vi "main-top-level-example.vi"() -> ()   [LabVIEW 2024]
uses:
  controls/digital-output-cluster.ctl
  controls/thermocouple-input-cluster.ctl
  controls/analog-input-cluster.ctl
  controls/adam-5000-cmd-response.ctl
  controls/state-enum.ctl
  controls/adam-5000-all-chassis-data.ctl
  controls/adam-5000-all-module-datas.ctl
  controls/digitial-input-cluster.ctl
  controls/analog-output-cluster.ctl
  controls/adam-5000-chassis-cmd-ack.ctl
  controls/adam-5000-chassis-module-types.ctl
  controls/adam-5000-DO-user-input.ctl
  controls/adam-5000-status-indicator-references.ctl
  controls/adam-5000-serial-settings.ctl
panel:
  out "Program State":T1
  in  "Start ADAM":bool
  out "cmd-response":T3
  out "Status Indicators":T4
  in  "Debug Mode":bool
  out "1.Thermocouple Inputs (degC)":T5
  in  "5:Digital Outputs":T6
  in  "4:Digital Outputs":T6
  out "0:Analog Inputs":T7
  out "3:Thermocouple Inputs (degC)":T5
  in  "Chassis Settings":T8={"VISA resource name"="COM8", "baud rate (19200)"=19200, "Chassis ID"=1}
  out "Loop Time (mS)":u32
  out "Loop Counter":i32
  out "error IO":errorcluster
  out "error":errorcluster
  in  "exit":bool
  # "ADAM 5000 Controller"
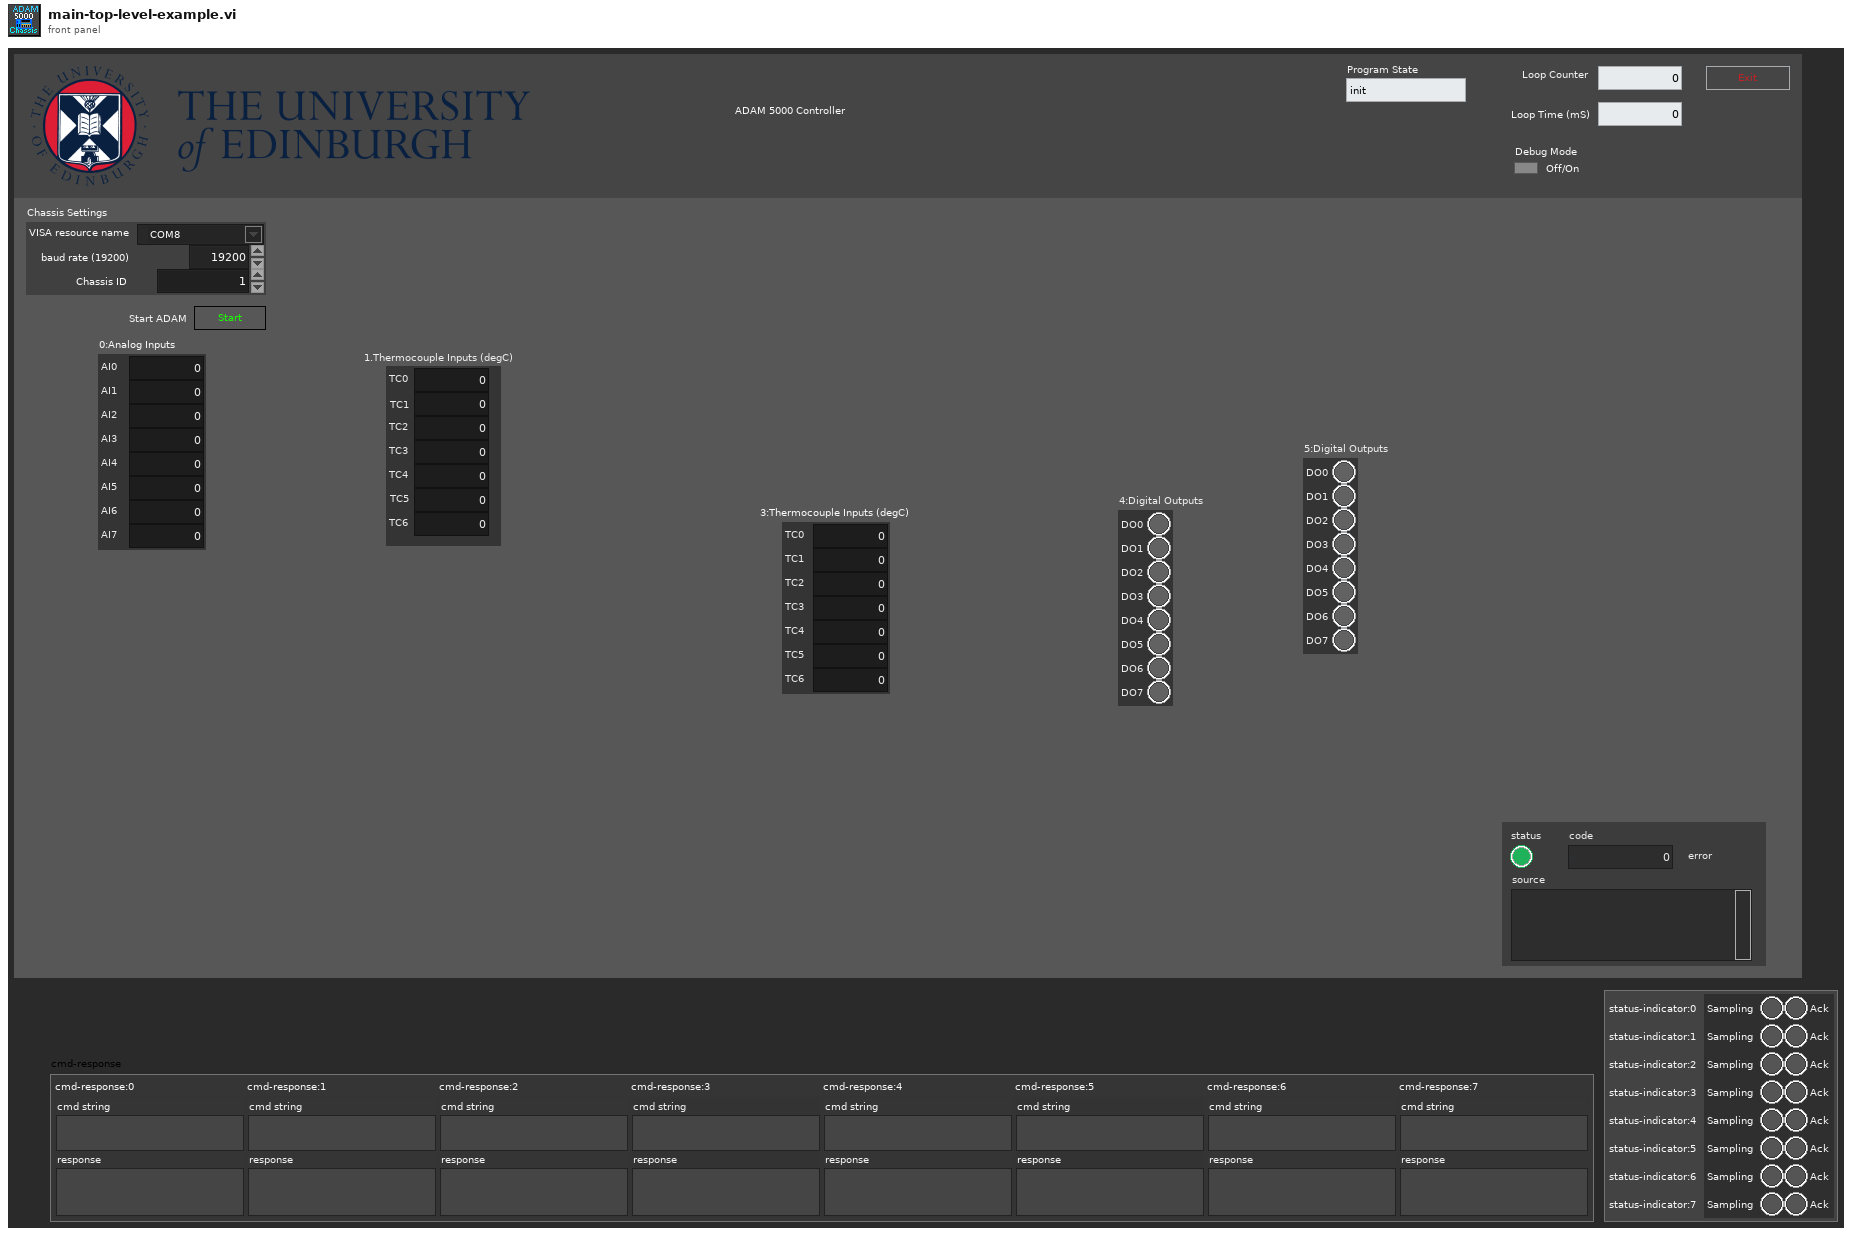
[diagram p1: front panel]
types:
  T1 = typedef "state-enum.ctl" = enum16{"init", "wait", "manual", "start", "run", "hold", "stop", "exit"}
  T2 = typedef "adam-5000-cmd-response.ctl" = cluster{"cmd string":string, "response":string}
  T3 = cluster{"cmd-response:0":T2, "cmd-response:1":T2, "cmd-response:2":T2, "cmd-response:3":T2, "cmd-response:4":T2, "cmd-response:5":T2, "cmd-response:6":T2, "cmd-response:7":T2}
  T4 = cluster{"status-indicator:0":cluster{"Sampling":bool, "Ack":bool}, "status-indicator:1":cluster{"Sampling":bool, "Ack":bool}, "status-indicator:2":cluster{"Sampling":bool, "Ack":bool}, "status-indicator:3":cluster{"Sampling":bool, "Ack":bool}, "status-indicator:4":cluster{"Sampling":bool, "Ack":bool}, "status-indicator:5":cluster{"Sampling":bool, "Ack":bool}, "status-indicator:6":cluster{"Sampling":bool, "Ack":bool}, "status-indicator:7":cluster{"Sampling":bool, "Ack":bool}}
  T5 = typedef "thermocouple-input-cluster.ctl" = cluster{"TC0":dbl, "TC1":dbl, "TC2":dbl, "TC3":dbl, "TC4":dbl, "TC5":dbl, "TC6":dbl}
  T6 = typedef "digital-output-cluster.ctl" = cluster{"DO0":bool, "DO1":bool, "DO2":bool, "DO3":bool, "DO4":bool, "DO5":bool, "DO6":bool, "DO7":bool}
  T7 = typedef "analog-input-cluster.ctl" = cluster{"AI0":dbl, "AI1":dbl, "AI2":dbl, "AI3":dbl, "AI4":dbl, "AI5":dbl, "AI6":dbl, "AI7":dbl}
  T8 = typedef "adam-5000-serial-settings.ctl" = cluster{"VISA resource name":refnum<visa-resource-name>, "baud rate (19200)":u32, "Chassis ID":u8}
  T9 = typedef "adam-5000-chassis-cmd-ack.ctl" = cluster{"cmd-response:0":T2, "cmd-response:1":T2, "cmd-response:2":T2, "cmd-response:3":T2, "cmd-response:4":T2, "cmd-response:5":T2, "cmd-response:6":T2, "cmd-response:7":T2}
  T10 = typedef "adam-5000-all-chassis-data.ctl" = cluster{"slot:0":T11, "slot:1":T11, "slot:2":T11, "slot:3":T11, "slot:4":T11, "slot:5":T11, "slot:6":T11, "slot:7":T11}
  T11 = typedef "adam-5000-all-module-datas.ctl" = cluster{"Digital Outputs":T6, "Digital Inputs":T12, "Analog Outputs":T13, "Analog Inputs":T7, "Thermocouple Inputs (degC)":T5}
  T12 = typedef "digitial-input-cluster.ctl" = cluster{"DI0":bool, "DI1":bool, "DI2":bool, "DI3":bool, "DI4":bool, "DI5":bool, "DI6":bool, "DI7":bool}
  T13 = typedef "analog-output-cluster.ctl" = cluster{"AO0":dbl, "AO1":dbl, "AO2":dbl, "AO3":dbl}
  T14 = enum16{"Digital Output", "Digital Input", "Analog Output", "Analog Input", "Thermocouple", "Power Relay", "empty"}
  T15 = enum8{"Enabled", "Disabled", "Disabled and Grayed Out"}
  T16 = typedef "adam-5000-status-indicator-references.ctl" = cluster{"status-indicator:0":refnum<vi>, "status-indicator:1":refnum<vi>, "status-indicator:2":refnum<vi>, "status-indicator:3":refnum<vi>, "status-indicator:4":refnum<vi>, "status-indicator:5":refnum<vi>, "status-indicator:6":refnum<vi>, "status-indicator:7":refnum<vi>}
  T17 = typedef "adam-5000-DO-user-input.ctl" = cluster{"0:Digital Outputs":T6, "1:Digital Outputs":T6, "2:Digital Outputs":T6, "3:Digital Outputs":T6, "4:Digital Outputs":T6, "5:Digital Outputs":T6, "6:Digital Outputs":T6, "7:Digital Outputs":T6}
  T18 = typedef "adam-5000-chassis-module-types.ctl" = cluster{"Slot 0: Module Type":enum16{"Digital Output", "Digital Input", "Analog Output", "Analog Input", "Thermocouple", "Power Relay", "empty"}, "Slot 1: Module Type":enum16{"Digital Output", "Digital Input", "Analog Output", "Analog Input", "Thermocouple", "Power Relay", "empty"}, "Slot 2: Module Type":enum16{"Digital Output", "Digital Input", "Analog Output", "Analog Input", "Thermocouple", "Power Relay", "empty"}, "Slot 3: Module Type":enum16{"Digital Output", "Digital Input", "Analog Output", "Analog Input", "Thermocouple", "Power Relay", "empty"}, "Slot 4: Module Type":enum16{"Digital Output", "Digital Input", "Analog Output", "Analog Input", "Thermocouple", "Power Relay", "empty"}, "Slot 5: Module Type":enum16{"Digital Output", "Digital Input", "Analog Output", "Analog Input", "Thermocouple", "Power Relay", "empty"}, "Slot 6: Module Type":enum16{"Digital Output", "Digital Input", "Analog Output", "Analog Input", "Thermocouple", "Power Relay", "empty"}, "Slot 7: Module Type":enum16{"Digital Output", "Digital Input", "Analog Output", "Analog Input", "Thermocouple", "Power Relay", "empty"}}
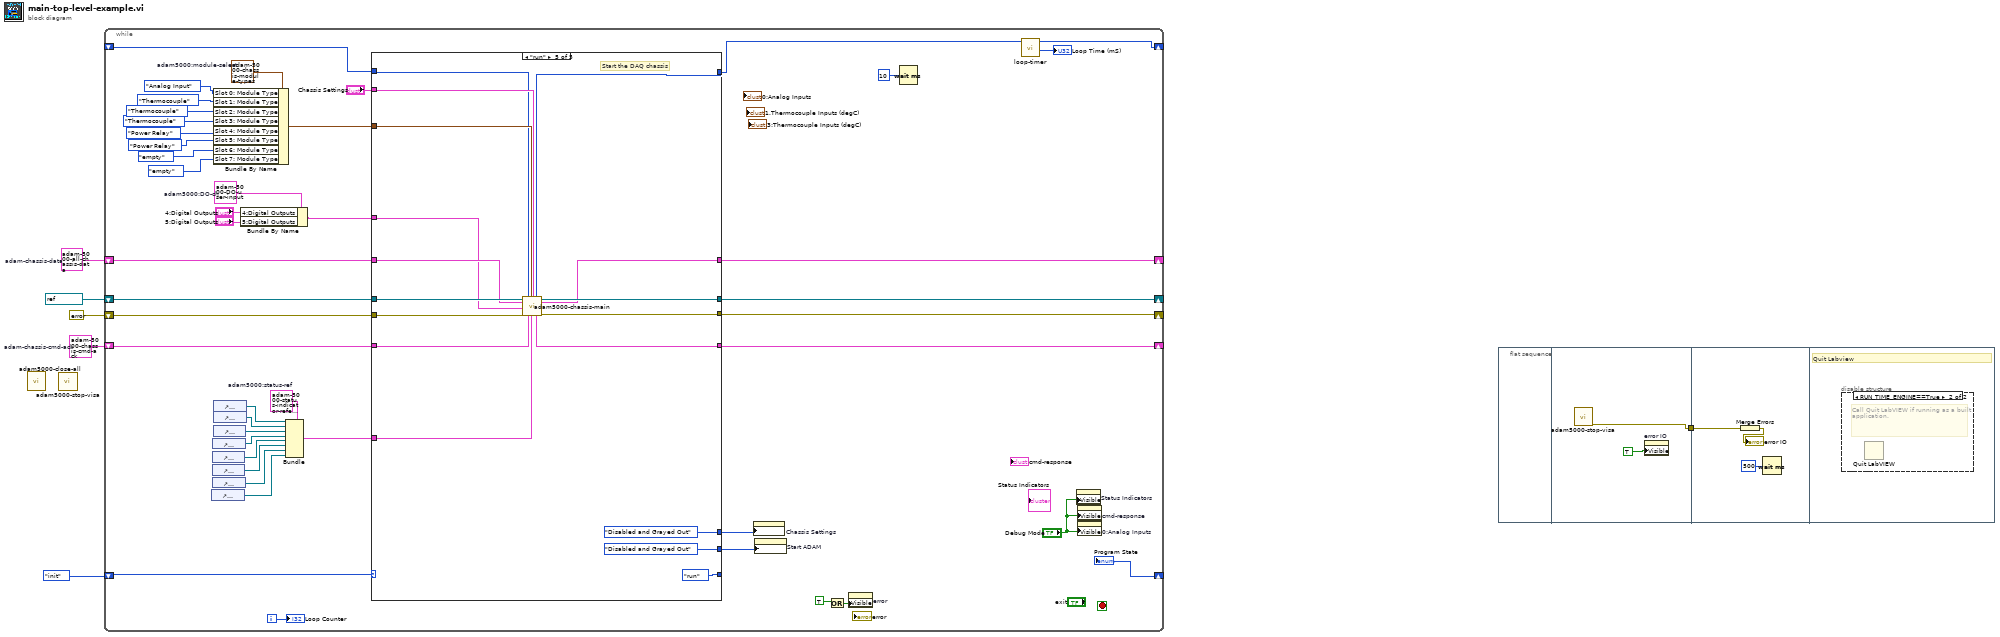
[diagram p0: block diagram]
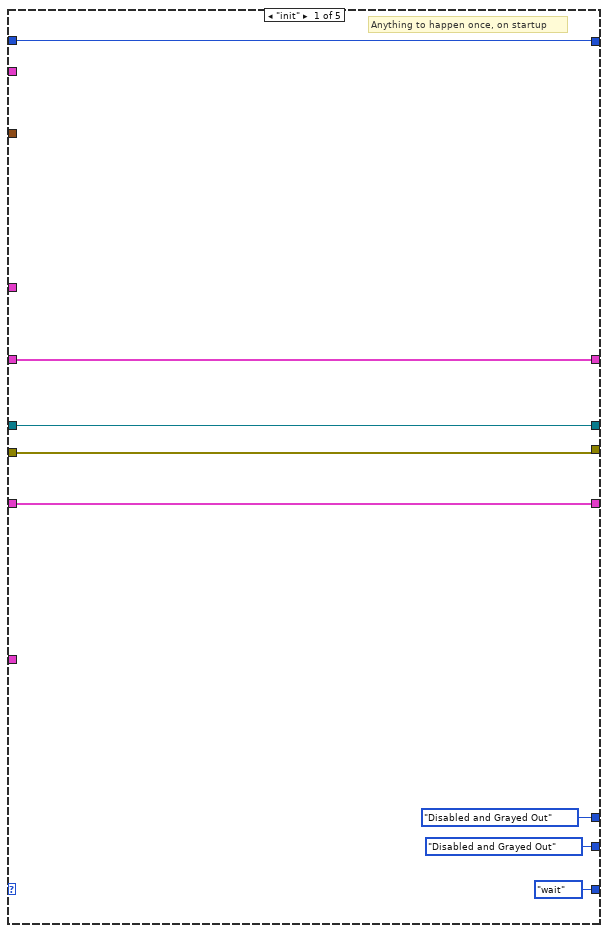
[diagram p3: hidden frame]
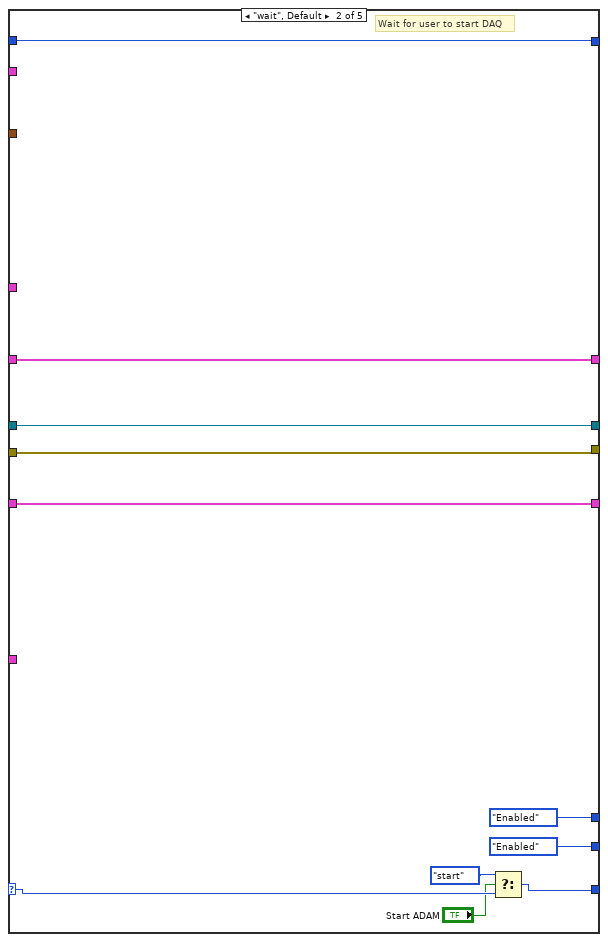
[diagram p4: hidden frame]
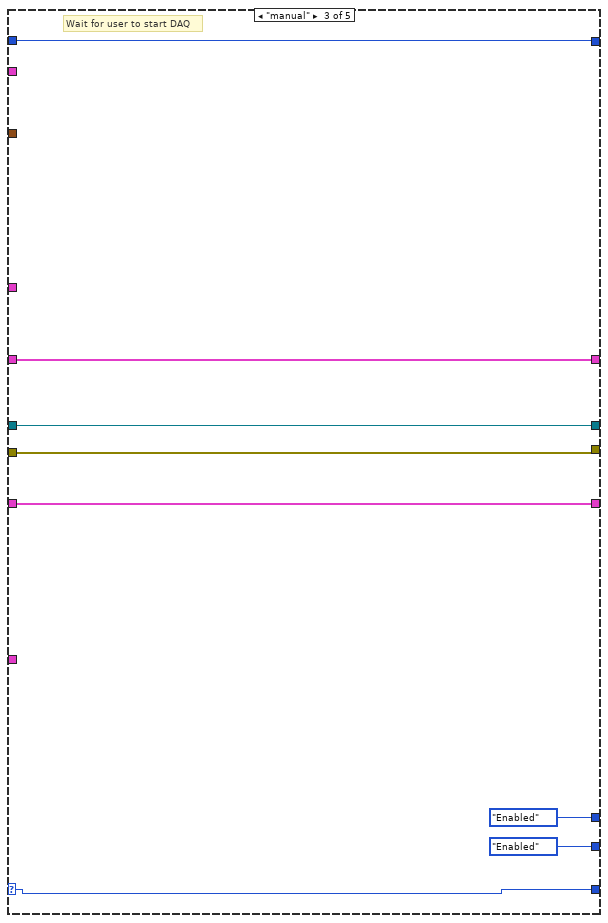
[diagram p5: hidden frame]
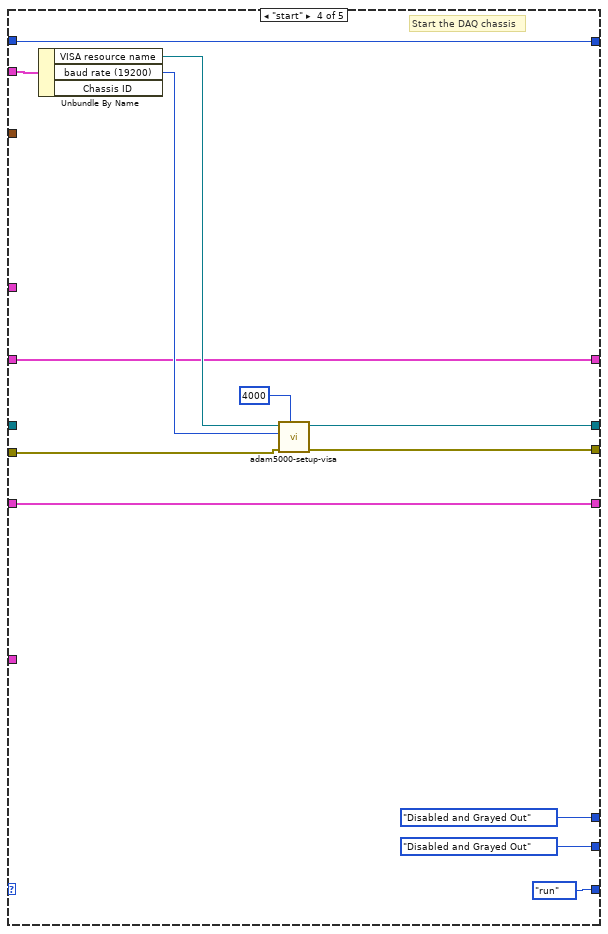
[diagram p6: hidden frame]
diagram:
  w1 = T9 {"cmd-response:0"={"cmd string"="", "response"=""}, "cmd-response:1"={"cmd string"="", "response"=""}, "cmd-response:2"={"cmd string"="", "response"=""}, "cmd-response:3"={"cmd string"="", "response"=""}, "cmd-response:4"={"cmd string"="", "response"=""}, "cmd-response:5"={"cmd string"="", "response"=""}, "cmd-response:6"={"cmd string"="", "response"=""}, "cmd-response:7"={"cmd string"="", "response"=""}}  # adam-chassis-cmd-ack
  w2 = T10 {"slot:0"={"Digital Outputs"={"DO0"=FALSE, "DO1"=FALSE, "DO2"=FALSE, "DO3"=FALSE, "DO4"=FALSE, "DO5"=FALSE, "DO6"=FALSE, "DO7"=FALSE}, "Digital Inputs"={"DI0"=FALSE, "DI1"=FALSE, "DI2"=FALSE, "DI3"=FALSE, "DI4"=FALSE, "DI5"=FALSE, "DI6"=FALSE, "DI7"=FALSE}, "Analog Outputs"={"AO0"=0.0, "AO1"=0.0, "AO2"=0.0, "AO3"=0.0}, "Analog Inputs"={"AI0"=0.0, "AI1"=0.0, "AI2"=0.0, "AI3"=0.0, "AI4"=0.0, "AI5"=0.0, "AI6"=0.0, "AI7"=0.0}, "Thermocouple Inputs (degC)"={"TC0"=0.0, "TC1"=0.0, "TC2"=0.0, "TC3"=0.0, "TC4"=0.0, "TC5"=0.0, "TC6"=0.0}}, "slot:1"={"Digital Outputs"={"DO0"=FALSE, "DO1"=FALSE, "DO2"=FALSE, "DO3"=FALSE, "DO4"=FALSE, "DO5"=FALSE, "DO6"=FALSE, "DO7"=FALSE}, "Digital Inputs"={"DI0"=FALSE, "DI1"=FALSE, "DI2"=FALSE, "DI3"=FALSE, "DI4"=FALSE, "DI5"=FALSE, "DI6"=FALSE, "DI7"=FALSE}, "Analog Outputs"={"AO0"=0.0, "AO1"=0.0, "AO2"=0.0, "AO3"=0.0}, "Analog Inputs"={"AI0"=0.0, "AI1"=0.0, "AI2"=0.0, "AI3"=0.0, "AI4"=0.0, "AI5"=0.0, "AI6"=0.0, "AI7"=0.0}, "Thermocouple Inputs (degC)"={"TC0"=0.0, "TC1"=0.0, "TC2"=0.0, "TC3"=0.0, "TC4"=0.0, "TC5"=0.0, "TC6"=0.0}}, "slot:2"={"Digital Outputs"={"DO0"=FALSE, "DO1"=FALSE, "DO2"=FALSE, "DO3"=FALSE, "DO4"=FALSE, "DO5"=FALSE, "DO6"=FALSE, "DO7"=FALSE}, "Digital Inputs"={"DI0"=FALSE, "DI1"=FALSE, "DI2"=FALSE, "DI3"=FALSE, "DI4"=FALSE, "DI5"=FALSE, "DI6"=FALSE, "DI7"=FALSE}, "Analog Outputs"={"AO0"=0.0, "AO1"=0.0, "AO2"=0.0, "AO3"=0.0}, "Analog Inputs"={"AI0"=0.0, "AI1"=0.0, "AI2"=0.0, "AI3"=0.0, "AI4"=0.0, "AI5"=0.0, "AI6"=0.0, "AI7"=0.0}, "Thermocouple Inputs (degC)"={"TC0"=0.0, "TC1"=0.0, "TC2"=0.0, "TC3"=0.0, "TC4"=0.0, "TC5"=0.0, "TC6"=0.0}}, "slot:3"={"Digital Outputs"={"DO0"=FALSE, "DO1"=FALSE, "DO2"=FALSE, "DO3"=FALSE, "DO4"=FALSE, "DO5"=FALSE, "DO6"=FALSE, "DO7"=FALSE}, "Digital Inputs"={"DI0"=FALSE, "DI1"=FALSE, "DI2"=FALSE, "DI3"=FALSE, "DI4"=FALSE, "DI5"=FALSE, "DI6"=FALSE, "DI7"=FALSE}, "Analog Outputs"={"AO0"=0.0, "AO1"=0.0, "AO2"=0.0, "AO3"=0.0}, "Analog Inputs"={"AI0"=0.0, "AI1"=0.0, "AI2"=0.0, "AI3"=0.0, "AI4"=0.0, "AI5"=0.0, "AI6"=0.0, "AI7"=0.0}, "Thermocouple Inputs (degC)"={"TC0"=0.0, "TC1"=0.0, "TC2"=0.0, "TC3"=0.0, "TC4"=0.0, "TC5"=0.0, "TC6"=0.0}}, "slot:4"={"Digital Outputs"={"DO0"=FALSE, "DO1"=FALSE, "DO2"=FALSE, "DO3"=FALSE, "DO4"=FALSE, "DO5"=FALSE, "DO6"=FALSE, "DO7"=FALSE}, "Digital Inputs"={"DI0"=FALSE, "DI1"=FALSE, "DI2"=FALSE, "DI3"=FALSE, "DI4"=FALSE, "DI5"=FALSE, "DI6"=FALSE, "DI7"=FALSE}, "Analog Outputs"={"AO0"=0.0, "AO1"=0.0, "AO2"=0.0, "AO3"=0.0}, "Analog Inputs"={"AI0"=0.0, "AI1"=0.0, "AI2"=0.0, "AI3"=0.0, "AI4"=0.0, "AI5"=0.0, "AI6"=0.0, "AI7"=0.0}, "Thermocouple Inputs (degC)"={"TC0"=0.0, "TC1"=0.0, "TC2"=0.0, "TC3"=0.0, "TC4"=0.0, "TC5"=0.0, "TC6"=0.0}}, "slot:5"={"Digital Outputs"={"DO0"=FALSE, "DO1"=FALSE, "DO2"=FALSE, "DO3"=FALSE, "DO4"=FALSE, "DO5"=FALSE, "DO6"=FALSE, "DO7"=FALSE}, "Digital Inputs"={"DI0"=FALSE, "DI1"=FALSE, "DI2"=FALSE, "DI3"=FALSE, "DI4"=FALSE, "DI5"=FALSE, "DI6"=FALSE, "DI7"=FALSE}, "Analog Outputs"={"AO0"=0.0, "AO1"=0.0, "AO2"=0.0, "AO3"=0.0}, "Analog Inputs"={"AI0"=0.0, "AI1"=0.0, "AI2"=0.0, "AI3"=0.0, "AI4"=0.0, "AI5"=0.0, "AI6"=0.0, "AI7"=0.0}, "Thermocouple Inputs (degC)"={"TC0"=0.0, "TC1"=0.0, "TC2"=0.0, "TC3"=0.0, "TC4"=0.0, "TC5"=0.0, "TC6"=0.0}}, "slot:6"={"Digital Outputs"={"DO0"=FALSE, "DO1"=FALSE, "DO2"=FALSE, "DO3"=FALSE, "DO4"=FALSE, "DO5"=FALSE, "DO6"=FALSE, "DO7"=FALSE}, "Digital Inputs"={"DI0"=FALSE, "DI1"=FALSE, "DI2"=FALSE, "DI3"=FALSE, "DI4"=FALSE, "DI5"=FALSE, "DI6"=FALSE, "DI7"=FALSE}, "Analog Outputs"={"AO0"=0.0, "AO1"=0.0, "AO2"=0.0, "AO3"=0.0}, "Analog Inputs"={"AI0"=0.0, "AI1"=0.0, "AI2"=0.0, "AI3"=0.0, "AI4"=0.0, "AI5"=0.0, "AI6"=0.0, "AI7"=0.0}, "Thermocouple Inputs (degC)"={"TC0"=0.0, "TC1"=0.0, "TC2"=0.0, "TC3"=0.0, "TC4"=0.0, "TC5"=0.0, "TC6"=0.0}}, "slot:7"={"Digital Outputs"={"DO0"=FALSE, "DO1"=FALSE, "DO2"=FALSE, "DO3"=FALSE, "DO4"=FALSE, "DO5"=FALSE, "DO6"=FALSE, "DO7"=FALSE}, "Digital Inputs"={"DI0"=FALSE, "DI1"=FALSE, "DI2"=FALSE, "DI3"=FALSE, "DI4"=FALSE, "DI5"=FALSE, "DI6"=FALSE, "DI7"=FALSE}, "Analog Outputs"={"AO0"=0.0, "AO1"=0.0, "AO2"=0.0, "AO3"=0.0}, "Analog Inputs"={"AI0"=0.0, "AI1"=0.0, "AI2"=0.0, "AI3"=0.0, "AI4"=0.0, "AI5"=0.0, "AI6"=0.0, "AI7"=0.0}, "Thermocouple Inputs (degC)"={"TC0"=0.0, "TC1"=0.0, "TC2"=0.0, "TC3"=0.0, "TC4"=0.0, "TC5"=0.0, "TC6"=0.0}}}  # adam-chassis-data
  n1 = call "adam5000-close-all.vi"() -> ()  [unwired: 12 in, 4 out]
  n2 = call "adam5000-stop-visa.vi"() -> ()  [unwired: 11 in, 1 out]
  n3 = while {
    shift-right: _ -> [w24]
    shift-left: state-enum."init" ("state-enum") -> [w25]
    shift-right: [w50] -> _
    shift-left: _ -> [w15]
    shift-right: [w20] -> _
    shift-left: refnum<visa-resource-name> "COM8" ("VISA Refnum out") -> [w21]
    shift-right: [w18] -> _
    shift-left: errorcluster {"status"=FALSE, "code"=0, "source"=""} ("error in") -> [w19]
    shift-right: [w8] -> _
    shift-left: w2 -> [w13]
    shift-right: [w9] -> _
    shift-left: w1 -> [w11]
    i -> [w51]
    stop <- _ stop-if-true
    w35 = T16 {"status-indicator:0"=refnum, "status-indicator:1"=refnum, "status-indicator:2"=refnum, "status-indicator:3"=refnum, "status-indicator:4"=refnum, "status-indicator:5"=refnum, "status-indicator:6"=refnum, "status-indicator:7"=refnum}  # adam5000:status-ref
    w38 = T17 {"0:Digital Outputs"={"DO0"=FALSE, "DO1"=FALSE, "DO2"=FALSE, "DO3"=FALSE, "DO4"=FALSE, "DO5"=FALSE, "DO6"=FALSE, "DO7"=FALSE}, "1:Digital Outputs"={"DO0"=FALSE, "DO1"=FALSE, "DO2"=FALSE, "DO3"=FALSE, "DO4"=FALSE, "DO5"=FALSE, "DO6"=FALSE, "DO7"=FALSE}, "2:Digital Outputs"={"DO0"=FALSE, "DO1"=FALSE, "DO2"=FALSE, "DO3"=FALSE, "DO4"=FALSE, "DO5"=FALSE, "DO6"=FALSE, "DO7"=FALSE}, "3:Digital Outputs"={"DO0"=FALSE, "DO1"=FALSE, "DO2"=FALSE, "DO3"=FALSE, "DO4"=FALSE, "DO5"=FALSE, "DO6"=FALSE, "DO7"=FALSE}, "4:Digital Outputs"={"DO0"=FALSE, "DO1"=FALSE, "DO2"=FALSE, "DO3"=FALSE, "DO4"=FALSE, "DO5"=FALSE, "DO6"=FALSE, "DO7"=FALSE}, "5:Digital Outputs"={"DO0"=FALSE, "DO1"=FALSE, "DO2"=FALSE, "DO3"=FALSE, "DO4"=FALSE, "DO5"=FALSE, "DO6"=FALSE, "DO7"=FALSE}, "6:Digital Outputs"={"DO0"=FALSE, "DO1"=FALSE, "DO2"=FALSE, "DO3"=FALSE, "DO4"=FALSE, "DO5"=FALSE, "DO6"=FALSE, "DO7"=FALSE}, "7:Digital Outputs"={"DO0"=FALSE, "DO1"=FALSE, "DO2"=FALSE, "DO3"=FALSE, "DO4"=FALSE, "DO5"=FALSE, "DO6"=FALSE, "DO7"=FALSE}}  # adam5000:DO-ch
    w39 = T18 {"Slot 0: Module Type"=enum."Digital Output", "Slot 1: Module Type"=enum."Digital Output", "Slot 2: Module Type"=enum."Digital Output", "Slot 3: Module Type"=enum."Digital Output", "Slot 4: Module Type"=enum."Digital Output", "Slot 5: Module Type"=enum."Digital Output", "Slot 6: Module Type"=enum."Digital Output", "Slot 7: Module Type"=enum."Digital Output"}  # adam5000:module-select
    n4 = control-ref of="status-indicator:7"() -> (w40:refnum<vi>)
    n5 = control-ref of="status-indicator:4"() -> (w43:refnum<vi>)
    n6 = control-ref of="status-indicator:5"() -> (w42:refnum<vi>)
    n7 = control-ref of="status-indicator:3"() -> (w44:refnum<vi>)
    n8 = control-ref of="status-indicator:6"() -> (w41:refnum<vi>)
    n9 = control-ref of="status-indicator:2"() -> (w45:refnum<vi>)
    n10 = Bundle By Name(cluster=w39, "Slot 0: Module Type"=T14."Analog Input", "Slot 1: Module Type"=T14."Thermocouple", "Slot 2: Module Type"=T14."Thermocouple" ("Slot 1: Module Type"), "Slot 3: Module Type"=T14."Thermocouple" ("Slot 1: Module Type"), "Slot 4: Module Type"=T14."Power Relay" ("Slot 1: Module Type"), "Slot 5: Module Type"=T14."Power Relay" ("Slot 1: Module Type"), "Slot 6: Module Type"=T14."empty" ("Slot 1: Module Type"), "Slot 7: Module Type"=T14."empty" ("Slot 1: Module Type")) -> (w16:T18)
    n11 = control-ref of="status-indicator:0"() -> (w47:refnum<vi>)
    n12 = control-ref of="status-indicator:1"() -> (w46:refnum<vi>)
    n13 = Bundle By Name(cluster=w38, "4:Digital Outputs"="4:Digital Outputs", "5:Digital Outputs"="5:Digital Outputs") -> (w12:T17)
    n14 = Bundle(cluster=w35, "status-indicator:0"=w47, "status-indicator:1"=w46, "status-indicator:2"=w45, "status-indicator:3"=w44, "status-indicator:4"=w43, "status-indicator:5"=w42, "status-indicator:6"=w41, "status-indicator:7"=w40) -> (w10:T16)
    n15 = case shown="\"run\"" w25 {
      selector: w25 -> [_ w69 w75 _ _]
      tunnel: [state-enum."wait" ("state-enum") w70 w75 state-enum."run" ("state-enum") state-enum."run" ("state-enum")] -> _
      tunnel: [T15."Disabled and Grayed Out" ("Disabled") T15."Enabled" ("Disabled") T15."Enabled" ("Disabled") T15."Disabled and Grayed Out" ("Disabled") T15."Disabled and Grayed Out" ("Disabled")] -> w23
      tunnel: [T15."Disabled and Grayed Out" ("Disabled") T15."Enabled" ("Disabled") T15."Enabled" ("Disabled") T15."Disabled and Grayed Out" ("Disabled") T15."Disabled and Grayed Out" ("Disabled")] -> w22
      tunnel: w21 -> [w57 w66 w77 _ w106]
      tunnel: [w57 w66 w77 w90 w104] -> w20
      tunnel: w19 -> [w56 w65 w76 w89 w105]
      tunnel: [w56 w65 w76 w88 w103] -> w18
      tunnel: "Chassis Settings" -> [_ _ _ w87 w102]
      tunnel: w16 -> [_ _ _ _ w101]
      tunnel: w15 -> [w55 w63 w74 w82 w100]
      tunnel: [w55 w63 w74 w82 w99] -> w14
      tunnel: w13 -> [w54 w62 w73 w81 w98]
      tunnel: w12 -> [_ _ _ _ w97]
      tunnel: w11 -> [w53 w61 w72 w80 w96]
      tunnel: w10 -> [_ _ _ _ w95]
      tunnel: [w53 w61 w72 w80 w94] -> w9
      tunnel: [w54 w62 w73 w81 w93] -> w8
      frame "init" {
        # "Anything to happen once, on startup"
      }
      frame "wait", Default {
        # "Wait for user to start DAQ"
        n16 = Select(t=state-enum."start" ("state-enum"), s="Start ADAM", f=w69) -> (s? t:f=w70:T1)
      }
      frame "manual" {
        # "Wait for user to start DAQ"
      }
      frame "start" {
        # "Start the DAQ chassis"
        n17 = Unbundle By Name(w87) -> ("VISA resource name"=w86:refnum<visa-resource-name>, "baud rate (19200)"=w85:u32)  [unwired: 1 out]
        n18 = call "adam5000-setup-visa.vi"("timeout (10sec)"=u32 4000, "error in"=w89, "baud rate (19200)"=w85, "VISA Refnum in"=w86) -> ("error out"=w88:errorcluster, "VISA Refnum out"=w90:refnum<visa-resource-name>)  [unwired: 6 in]
      }
      frame "run" {
        # "Start the DAQ chassis"
        n19 = call "adam5000-chassis-main.vi"("VISA Refnum In"=w106, "adam-chassis-all-data-in"=w98, "adam-chassis-all-DO-in"=w97, "error in"=w105, "loop-time-in"=w100, "adam-chassis-cmd-response-in"=w96, "adam-chassis-module-select-in"=w101, "adam5000:status-ref-in"=w95, "Chassis Settings"=w102) -> ("loop-time-out"=w99:u32, "adam-chassis-cmd-response-out"=w94:T9, "VISA Refnum Out"=w104:refnum<visa-resource-name>, "adam-chassis-all-data-out"=w93:T10, "error out"=w103:errorcluster)  [unwired: 5 in, 1 out]
      }
    }
    n20 = property on="Chassis Settings" class="Clust (strict)"("DisabledEnum"=w23) -> ()  [unwired: 2 in, 2 out]
    n21 = property on="Start ADAM" class="Bool"("DisabledEnum"=w22) -> ()  [unwired: 2 in, 2 out]
    n22 = Or(x=TRUE ("Debug Mode")) -> (x .or. y?=w49:bool)  [unwired: 1 in]
    n23 = property on="error" class="Clust (strict)"("Visible"=w49) -> ()  [unwired: 2 in, 2 out]
    n24 = Wait (ms)(milliseconds to wait=u32 10) -> ()  [unwired: 1 out]
    n25 = call "loop-timer.vi"("loop-time-in"=w14) -> ("Loop Time (mS)"=→"Loop Time (mS)":u32, "loop-time-out"=w50:u32)  [unwired: 9 in]
    n26 = property on="Status Indicators" class="Clust (strict)"("Visible"="Debug Mode") -> ()  [unwired: 2 in, 2 out]
    n27 = property on="cmd-response" class="Clust (strict)"("Visible"="Debug Mode") -> ()  [unwired: 2 in, 2 out]
    n28 = property on="0:Analog Inputs" class="Clust (strict)"("Visible"="Debug Mode") -> ()  [unwired: 2 in, 2 out]
    "Loop Counter" <- w51
    "Program State" <- w24
  }
  n29 = flat-sequence {
    tunnel: [w110] -> w5
    tunnel: w5 -> [w112]
    frame #0 {
    }
    frame #1 {
      n30 = call "adam5000-stop-visa.vi"() -> ("error out"=w110:errorcluster)  [unwired: 11 in]
      n31 = property on="error IO" class="Clust (strict)"("Visible"=TRUE) -> ()  [unwired: 2 in, 2 out]
    }
    frame #2 {
      n32 = Merge Errors(w112) -> (→"error IO":errorcluster)
      n33 = Wait (ms)(milliseconds to wait=u32 500) -> ()  [unwired: 1 out]
    }
    frame #3 {
      # "Quit Labview"
      n34 = disable-structure "Conditional Disable Structure" shown="RUN_TIME_ENGINE==True" {
        frame condition #0 (active) {
        }
        frame condition #1 {
          # "Call Quit LabVIEW if running as a built application."
          n35 = Quit LabVIEW() -> ()  [unwired: 1 in]
        }
      }
    }
  }
